vi "_Green Bars.vi"() -> (3 "Green Bars":T1[](array[typedef])=[{"image type"=0, "image depth"=32, "image"=array[151360 elements], "mask"=array[4816 elements], "colors"=[], "Rectangle"={"left"=0, "top"=0, "right"=220, "bottom"=172}}, {"image type"=0, "image depth"=32, "image"=array[151360 elements], "mask"=array[4816 elements], "colors"=[], "Rectangle"={"left"=0, "top"=0, "right"=220, "bottom"=172}}, {"image type"=0, "image depth"=32, "image"=array[151360 elements], "mask"=array[4816 elements], "colors"=[], "Rectangle"={"left"=0, "top"=0, "right"=220, "bottom"=172}}, {"image type"=0, "image depth"=32, "image"=array[151360 elements], "mask"=array[4816 elements], "colors"=[], "Rectangle"={"left"=0, "top"=0, "right"=220, "bottom"=172}}, {"image type"=0, "image depth"=32, "image"=array[151360 elements], "mask"=array[4816 elements], "colors"=[], "Rectangle"={"left"=0, "top"=0, "right"=220, "bottom"=172}}, {"image type"=0, "image depth"=32, "image"=array[151360 elements], "mask"=array[4816 elements], "colors"=[], "Rectangle"={"left"=0, "top"=0, "right"=220, "bottom"=172}}, {"image type"=0, "image depth"=32, "image"=array[151360 elements], "mask"=array[4816 elements], "colors"=[], "Rectangle"={"left"=0, "top"=0, "right"=220, "bottom"=172}}, {"image type"=0, "image depth"=32, "image"=array[151360 elements], "mask"=array[4816 elements], "colors"=[], "Rectangle"={"left"=0, "top"=0, "right"=220, "bottom"=172}}])   [LabVIEW 2011, in "LVH-Build-Tools.lvlib"]
uses:
  <vilib>/picture/picture.llb/imagedata.ctl
  LVH-Build-Tools.lvlib
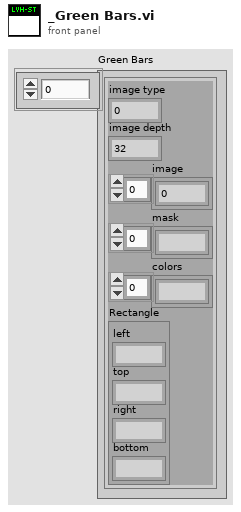
[diagram p1: front panel]
types:
  T1 = typedef "imagedata.ctl" = cluster{"image type":i32, "image depth":i32, "image":u8[], "mask":u8[], "colors":u32[], "Rectangle":cluster{"left":i16, "top":i16, "right":i16, "bottom":i16}}
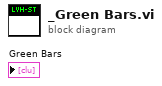
[diagram p0: block diagram]
diagram:
